vi "LogActuators.vi"(8 "error in (no error)":errorcluster, 11 "All actuators":T1) -> (0 "error out":errorcluster, 3 "spreadsheet string":string)   [LabVIEW 2015]
uses:
  <vilib>/Rock Robotics/WPI/CAN/Jaguar/SubVIs/WPI_CANJaguar_ControlMode.ctl
  <vilib>/Rock Robotics/WPI/CAN/TalonSRX/WPI_CANTalonSRX_APIControlMode.ctl
  <vilib>/Rock Robotics/SystemInterfaces/DIO/FPGA_DIOPWMChannel.ctl
  <vilib>/Rock Robotics/WPI/PWM/WPI_PWMDeadband.ctl
  <vilib>/Rock Robotics/WPI/MotorControl/WPI_MotorControlType.ctl
  <vilib>/Rock Robotics/WPI/MotorControl/WPI_MotorControlDeviceRef.ctl
  <vilib>/Rock Robotics/WPI/RobotDrive/WPI_RobotDriveDevRef.ctl
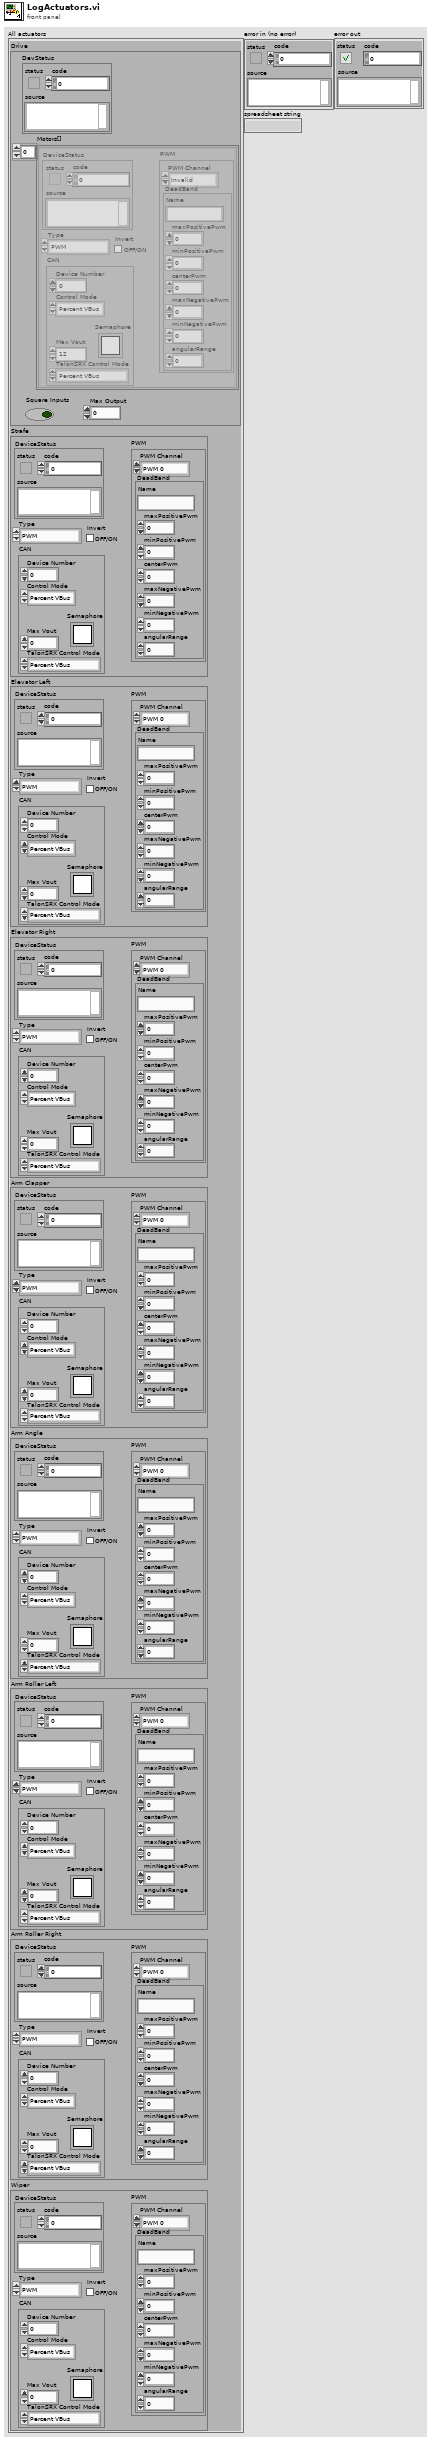
[diagram p1: front panel]
types:
  T1 = typedef "Actuators.ctl" = cluster{"Drive":T2, "Strafe":T3, "Elevator Left":T3, "Elevator Right":T3, "Arm Clapper":T3, "Arm Angle":T3, "Arm Roller Left":T3, "Arm Roller Right":T3, "Wiper":T3}
  T2 = typedef "WPI_RobotDriveDevRef.ctl" = cluster{"DevStatus":errorcluster, "Motors[]":T3[], "Square Inputs":bool, "Max Output":dbl}
  T3 = typedef "WPI_MotorControlDeviceRef.ctl" = cluster{"DeviceStatus":errorcluster, "Type":T4, "PWM":cluster{"PWM Channel":T5, "DeadBand":T6}, "CAN":cluster{"Device Number":u8, "Control Mode":T7, "Semaphore":T8, "Max Vout":dbl, "TalonSRX Control Mode":T9}, "Invert":bool}
  T4 = typedef "WPI_MotorControlType.ctl" = enum16{"PWM", "CAN", "CANTalonSRX"}
  T5 = typedef "FPGA_DIOPWMChannel.ctl" = enum8{"PWM 0", "PWM 1", "PWM 2", "PWM 3", "PWM 4", "PWM 5", "PWM 6", "PWM 7", "PWM 8", "PWM 9", "PWM MXP 0", "PWM MXP 1", "PWM MXP 2", "PWM MXP 3", "PWM MXP 4", "PWM MXP 5", "PWM MXP 6", "PWM MXP 7", "PWM MXP 8", "PWM MXP 9", "Invalid"}
  T6 = typedef "WPI_PWMDeadband.ctl" = cluster{"Name":string, "maxPositivePwm":i32, "minPositivePwm":i32, "centerPwm":i32, "maxNegativePwm":i32, "minNegativePwm":i32, "angularRange":u16}
  T7 = typedef "WPI_CANJaguar_ControlMode.ctl" = enum8{"Percent VBus", "Current", "Speed", "Position", "Voltage"}
  T8 = typedef "Semaphore RefNum" = refnum<k1>
  T9 = typedef "WPI_CANTalonSRX_APIControlMode.ctl" = enum8{"Percent VBus", "Speed", "Position", "Slave", "Unchanged / Invalid", "Voltage Compensation", "Current", "Motion Profile"}
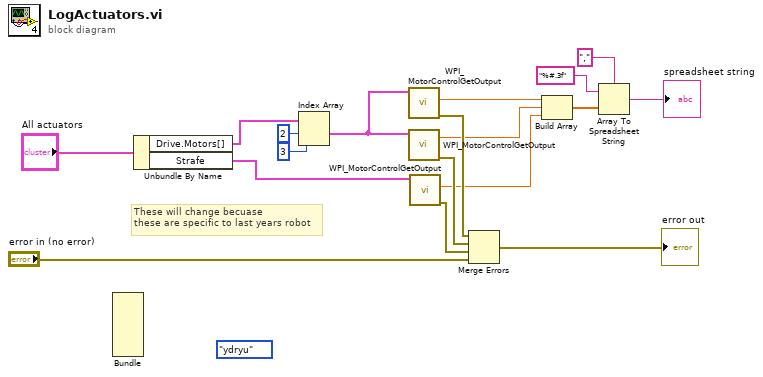
[diagram p0: block diagram]
diagram:
  (unwired) enum16{"ydryu"}."ydryu"
  # "These will change becuase\nthese are specific to last years robot"
  n1 = Bundle() -> ()  [unwired: 9 in, 1 out]
  n2 = Unbundle By Name("All actuators") -> ("Drive.Motors[]"=w18:T3[], "Strafe"=w14:T3)
  n3 = Index Array(array=w18, index #1=2 ("index"), index #2=3 ("index")) -> (element #1=w15:T3)  [unwired: 1 out]
  n4 = call <vilib>:"WPI_MotorControlGetOutput.vi"("MotorControlDevRef"=w15) -> ("error out"=w10:errorcluster, "Output"=w9:dbl)  [unwired: 8 in, 1 out]
  n5 = call <vilib>:"WPI_MotorControlGetOutput.vi"("MotorControlDevRef"=w15) -> ("error out"=w11:errorcluster, "Output"=w8:dbl)  [unwired: 8 in, 1 out]
  n6 = call <vilib>:"WPI_MotorControlGetOutput.vi"("MotorControlDevRef"=w14) -> ("error out"=w13:errorcluster, "Output"=w7:dbl)  [unwired: 8 in, 1 out]
  n7 = Merge Errors(w10, w11, w13, "error in (no error)") -> (→"error out":errorcluster)
  n8 = Build Array(w9, w8, w7) -> (w6:dbl[])
  n9 = Array To Spreadsheet String(delimiter (Tab)=",", array=w6, 3:"%#.3f" ("format string")) -> (spreadsheet string=→"spreadsheet string":string)
